vi "AddandUpdateUsers.vi"() -> ()   [LabVIEW 2017]
uses:
  User_cluster.ctl
  DatabaseContollerGFVenum.ctl
  <vilib>/addons/Database/_DB Variant To Data/Database Variant To Data.xnode
panel:
  in  "Surname":string
  in  "Cancel Button":bool
  in  "Load \nImage \n(JPG )":path
  in  "CreateUser Button":bool
  in  "Save Button":bool
  out "User Picture":T1(plugin-control)
  in  "Active Checkbox":bool
  out "Index":i32
  in  "Affiliation":string
  in  "Phone":string
  in  "Title":string
  in  "Password":string
  in  "Name":string
  in  "Users ListBox":i32(listbox)
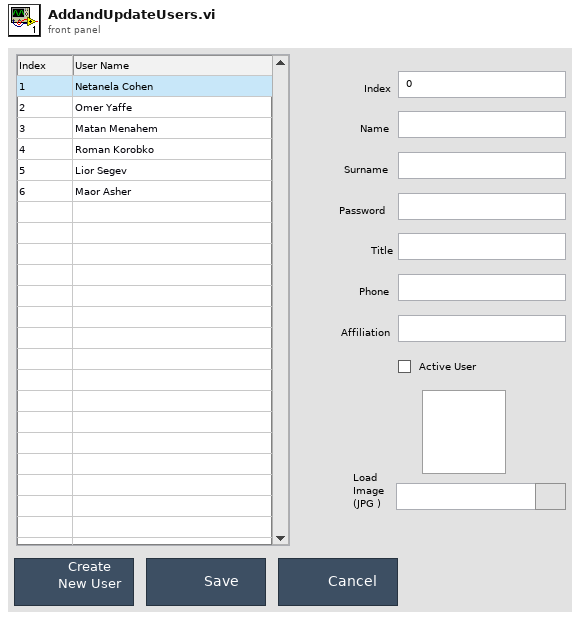
[diagram p1: front panel]
types:
  T1 = typedef "IMAQ Image.ctl" = refnum<image>
  T2 = typedef "User_cluster.ctl" = cluster{"Index":dbl, "Name":string, "Surname":string, "Password":string, "Title":string, "Phone":string, "Affiliation":string, "Active User":bool, "User Image":string}
  T3 = typedef "DatabaseContollerGFVenum.ctl" = enum16{"Init and Open Database!", "GetUserData!", "GetUsersAllTable!", "GetTimeDifferencebetweenLastTwoMeasurements!", "Get next Journal Number!", "WriteInJournalTable", "GetNewMeas_dataIndex", "UpdateWithSpectrometerData", "UpdateWithMicroscopeData", "UpdateWithMapScriptData", "UpdateWithmainUIData", "Get Objective Microns/Pixels", "Get User Name!", "Get Active Users Names!", "Get User Picture!", "Get User Phone Number!", "Get Setup Names!", "Get Active Microscope Objectives!", "Get Experiment Number!", "Get Sample Types!", "Write meas_conf Table", "Write meas_data Table", "GetListOfIndices", "Get Objective Index", "Get last X Journal Entries"}
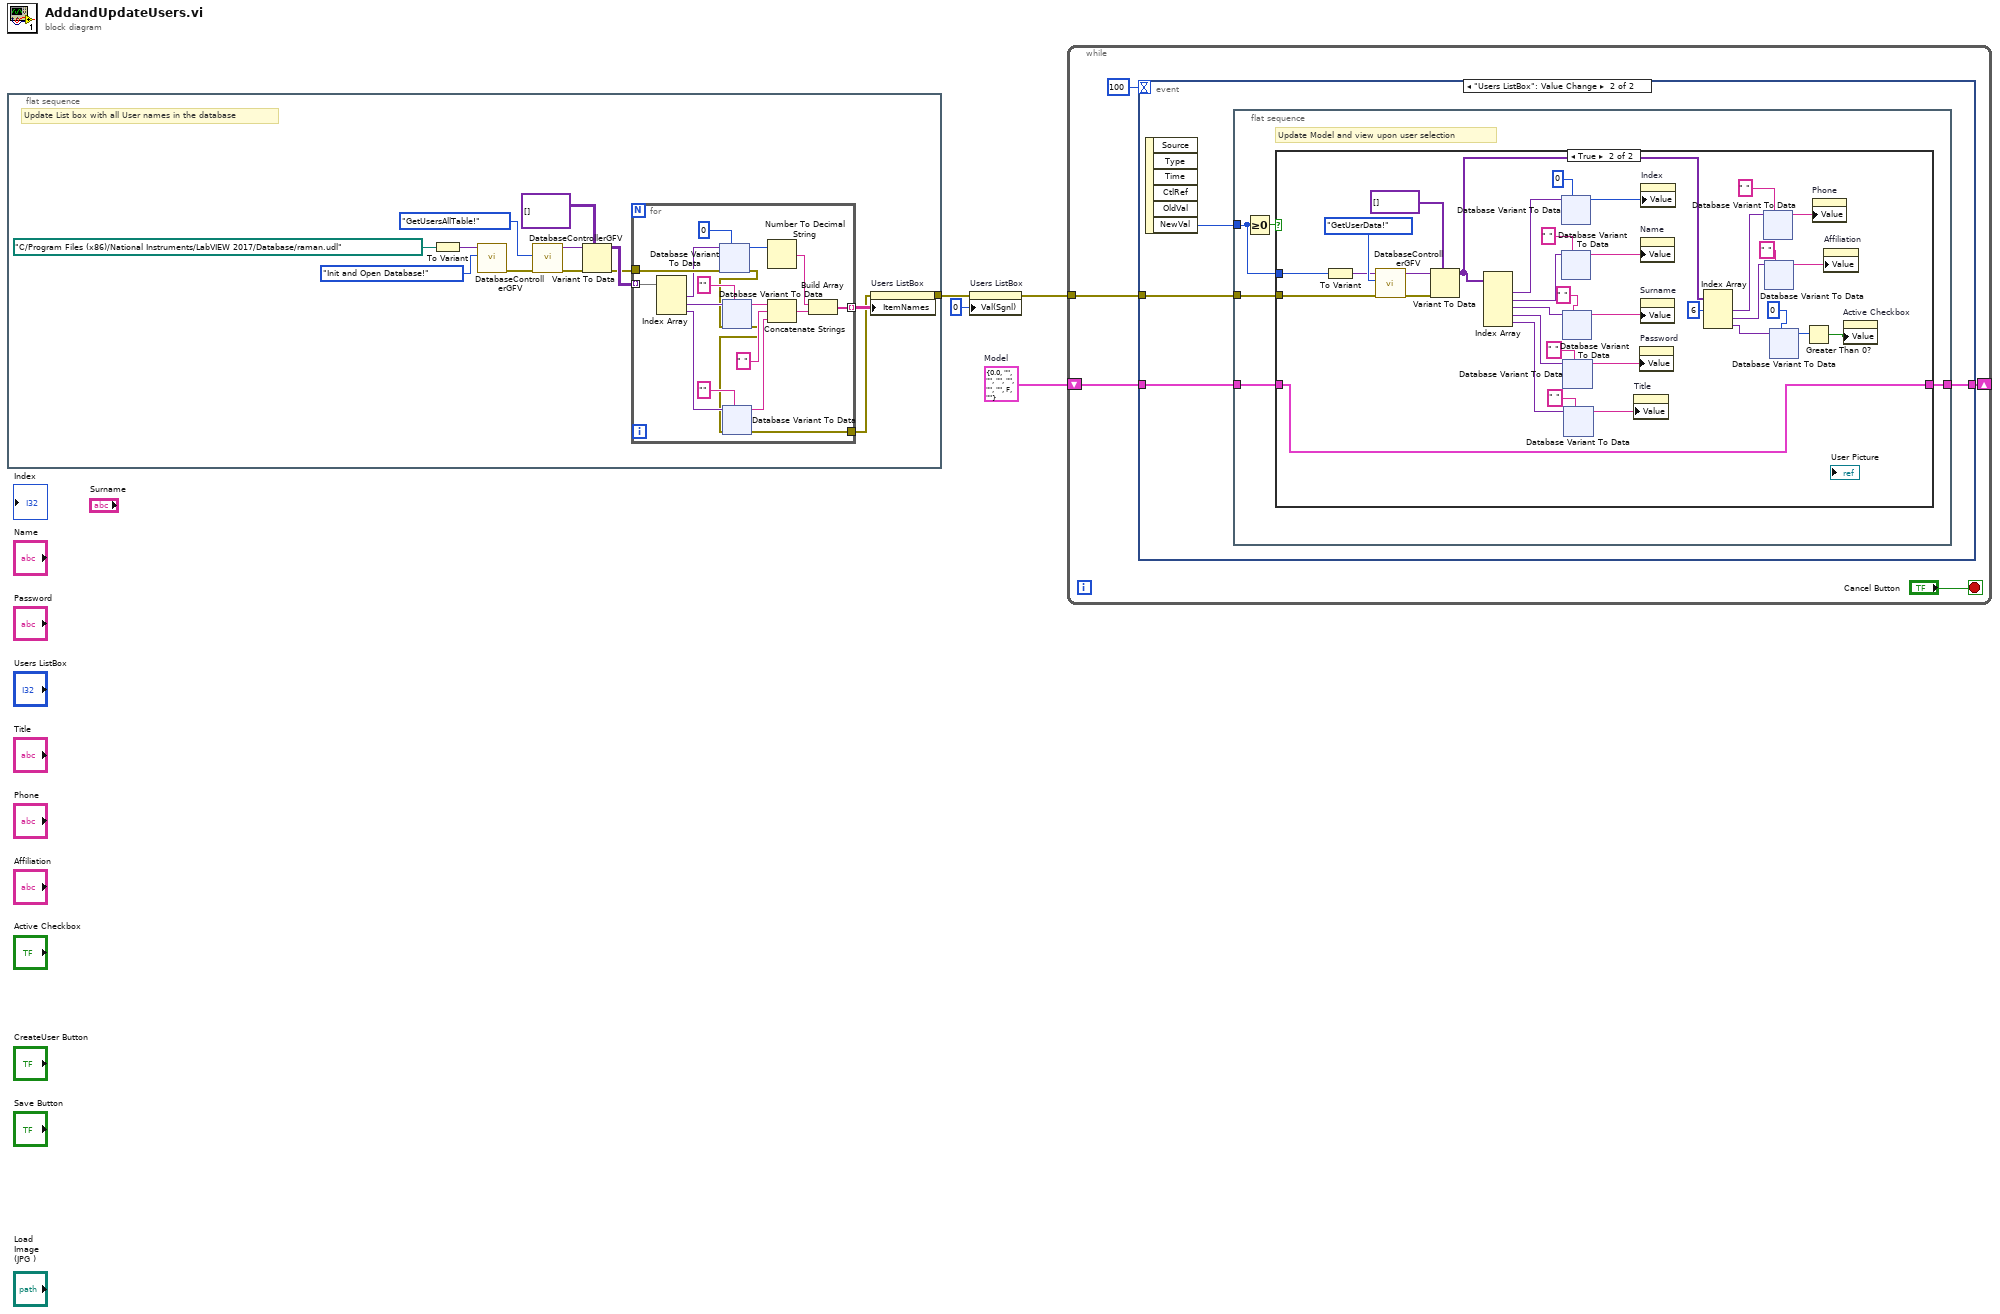
[diagram p0: block diagram]
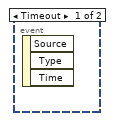
[diagram p2: hidden frame]
diagram:
  w1 = T2 {"Index"=0.0, "Name"="", "Surname"="", "Password"="", "Title"="", "Phone"="", "Affiliation"="", "Active User"=FALSE, "User Image"=""}  # Model
  n1 = flat-sequence {
    tunnel: [w5] -> w4
    frame #0 {
      # "Update List box with all User names in the database"
      n2 = To Variant(anything=path "C:/Program Files (x86)/National Instruments/LabVIEW 2017/Database/raman.udl" ("connection information")) -> (Variant=w16:variant)
      n3 = call "DatabaseControllerGFV.vi"("Enum"=DatabaseContollerGFVenum."Init and Open Database!", "Data in"=w16) -> ("error out"=w14:errorcluster)  [unwired: 8 in, 1 out]
      n4 = call "DatabaseControllerGFV.vi"("error in (no error)"=w14, "Enum"=DatabaseContollerGFVenum."GetUsersAllTable!") -> ("error out"=w12:errorcluster, "Data Out"=w11:variant)  [unwired: 8 in]
      n5 = Variant To Data(error in=w12, type=variant[][] [] ("data"), Variant=w11) -> (data=w9:variant[][], error out=w8:errorcluster)
      n6 = for {
        tunnel: w9 -> [w34] mode=indexing
        tunnel: w8 -> [w35]
        tunnel: [w23] -> w7 mode=indexing
        tunnel: [w18] -> w6
        n7 = Index Array(array=w34) -> (element #1=w33:variant, element #2=w31:variant, element #3=w28:variant)  [unwired: 3 in]
        n8 = xnode "Database Variant To Data"("database variant"=w33, "error in (no error)"=w35, "type"=0) -> ("data"=w26:i32, "error out"=w20:errorcluster)
        n9 = xnode "Database Variant To Data"("database variant"=w31, "error in (no error)"=w20, "type"="") -> ("data"=w22:string, "error out"=w19:errorcluster)
        n10 = xnode "Database Variant To Data"("database variant"=w28, "error in (no error)"=w19, "type"="") -> ("data"=w21:string, "error out"=w18:errorcluster)
        n11 = Number To Decimal String(number=w26) -> (decimal integer string=w25:string)  [unwired: 1 in]
        n12 = Concatenate Strings(w22, " " ("string"), w21) -> (w24:string)
        n13 = Build Array(w25, w24) -> (w23:string[])
      }
      n14 = property on="Users ListBox" class="MCListbox (strict)"(error in=w6, "ItemNames"=w7) -> (error out=w5:errorcluster)  [unwired: 1 in, 1 out]
    }
  }
  n15 = property on="Users ListBox" class="MCListbox (strict)"(error in=w4, "Val(Sgnl)"=0 ("Value (Signaling)")) -> (error out=w2:errorcluster)  [unwired: 1 in, 1 out]
  n16 = while {
    tunnel: w2 -> [w133]
    shift-right: [w132] -> _
    shift-left: w1 -> [w134]
    stop <- "Cancel Button" stop-if-true
    n17 = event shown="[1] \"Users ListBox\": Value Change" {
      selector: _ -> [_ _]
      dyn-events: _ -> [_ _]
      timeout: 100 -> [_ _]
      tunnel: w134 -> [_ w139]
      tunnel: w133 -> [_ w138]
      tunnel: [_ w137] -> w132
      event Timeout {
        n18 = event-data() -> ()  [unwired: 1 in, 3 out]
      }
      event "Users ListBox": Value Change {
        n19 = event-data() -> ("NewVal"=w140:i32)  [unwired: 1 in, 5 out]
        n20 = flat-sequence {
          tunnel: w140 -> [w142]
          tunnel: w139 -> [w144]
          tunnel: w138 -> [w143]
          tunnel: [w141] -> w137
          frame #0 {
            # "Update Model and view upon user selection"
            n21 = Greater Or Equal To 0?(x=w142) -> (x >= 0?=w145:bool)
            n22 = case shown="True" w145 {
              tunnel: w144 -> [w146 w150]
              tunnel: w143 -> [_ w181]
              tunnel: w142 -> [_ w178]
              tunnel: [w146 w150] -> w141
              frame False {
              }
              frame True {
                n23 = To Variant(anything=w178) -> (Variant=w179:variant)
                n24 = call "DatabaseControllerGFV.vi"("error in (no error)"=w181, "Enum"=DatabaseContollerGFVenum."GetUserData!", "Data in"=w179) -> ("error out"=w177:errorcluster, "Data Out"=w176:variant)  [unwired: 7 in]
                n25 = Variant To Data(error in=w177, type=variant[] [] ("subarray"), Variant=w176) -> (data=w159:variant[])  [unwired: 1 out]
                n26 = Index Array(array=w159) -> (element #1=w174:variant, element #2=w171:variant, element #3=w168:variant, element #4=w164:variant, element #5=w161:variant)  [unwired: 5 in]
                n27 = xnode "Database Variant To Data"("database variant"=w174, "type"=0 ("NewVal")) -> ("data"=w172:i32)  [unwired: 1 in, 1 out]
                n28 = xnode "Database Variant To Data"("database variant"=w171, "type"=" " ("string")) -> ("data"=w169:string)  [unwired: 1 in, 1 out]
                n29 = xnode "Database Variant To Data"("database variant"=w168, "type"=" " ("string")) -> ("data"=w166:string)  [unwired: 1 in, 1 out]
                n30 = xnode "Database Variant To Data"("database variant"=w164, "type"=" " ("string")) -> ("data"=w163:string)  [unwired: 1 in, 1 out]
                n31 = xnode "Database Variant To Data"("database variant"=w161, "type"=" " ("string")) -> ("data"=w160:string)  [unwired: 1 in, 1 out]
                n32 = property on="Title" class="Str"("Value"=w160) -> ()  [unwired: 2 in, 2 out]
                n33 = property on="Password" class="Str"("Value"=w163) -> ()  [unwired: 2 in, 2 out]
                n34 = property on="Name" class="Str"("Value"=w169) -> ()  [unwired: 2 in, 2 out]
                n35 = property on="Surname" class="Str"("Value"=w166) -> ()  [unwired: 2 in, 2 out]
                n36 = property on="Index" class="DigNum (strict)"("Value"=w172) -> ()  [unwired: 2 in, 2 out]
                n37 = Index Array(array=w159, index #1=6 ("index")) -> (element #1=w157:variant, element #2=w154:variant, element #3=w151:variant)  [unwired: 2 in]
                n38 = xnode "Database Variant To Data"("database variant"=w157, "type"=" " ("string")) -> ("data"=w155:string)  [unwired: 1 in, 1 out]
                n39 = xnode "Database Variant To Data"("database variant"=w154, "type"=" " ("string")) -> ("data"=w152:string)  [unwired: 1 in, 1 out]
                n40 = xnode "Database Variant To Data"("database variant"=w151, "type"=0 ("NewVal")) -> ("data"=w148:i32)  [unwired: 1 in, 1 out]
                n41 = Greater Than 0?(x=w148) -> (x > 0?=w147:bool)
                n42 = property on="Phone" class="Str"("Value"=w155) -> ()  [unwired: 2 in, 2 out]
                n43 = property on="Affiliation" class="Str"("Value"=w152) -> ()  [unwired: 2 in, 2 out]
                n44 = property on="Active Checkbox" class="Bool (strict)"("Value"=w147) -> ()  [unwired: 2 in, 2 out]
              }
            }
          }
        }
      }
    }
  }
